vi "analysis_01(SubVI).vi"(8 "에러 입력(에러 없음)":errorcluster, 10 "품   번":string="034220", 11 "참조 번호 입력":T1 caption="client handle out") -> (0 "에러 출력":errorcluster, 1 "거래량":waveform(dbl)(graph), 2 "가격":waveform(i32)(graph), 3 "참조 번호 출력":T1 caption="client handle out", 5 "출력":T2)   [LabVIEW 2018]
uses:
  <vilib>/httpClient/ClientHandle.ctl
  <vilib>/httpClient/LabVIEWHTTPClient.lvlib
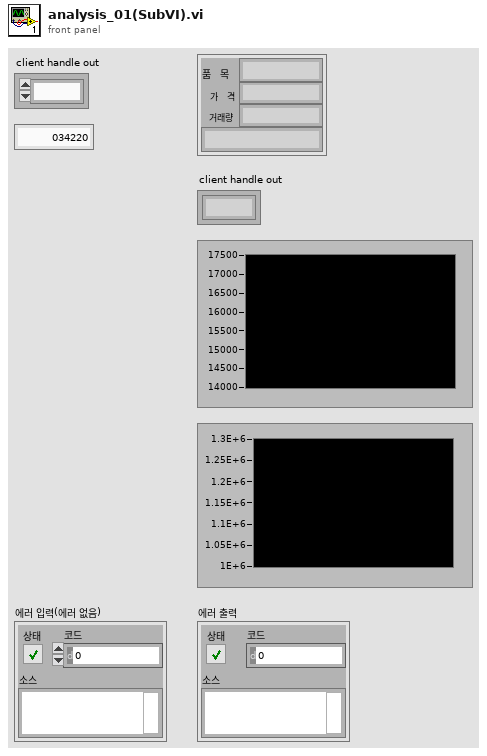
[diagram p1: front panel]
types:
  T1 = typedef "LabVIEWHTTPClient.lvlib/ClientHandle.ctl" = refnum<k1>
  T2 = cluster{"품   목":string, "가   격":i32, "거래량":dbl, "일시":string}
  T3 = cluster{"품목":string, "가격":i32, "거래량":dbl, "일시":string}
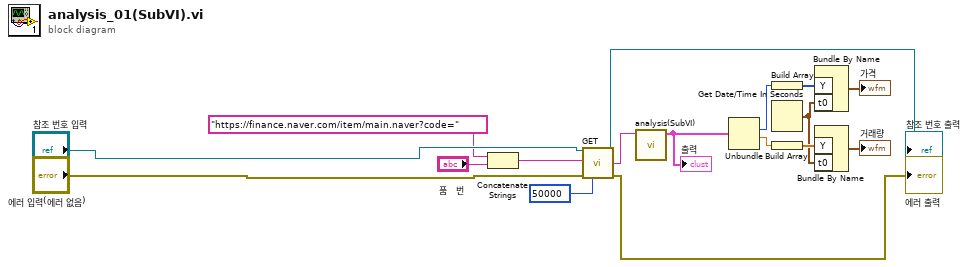
[diagram p0: block diagram]
diagram:
  n1 = Concatenate Strings("https://finance.naver.com/item/main.naver?code=" ("url"), "품   번") -> (w1:string)
  n2 = call <vilib>:"GET.vi"("client handle"="참조 번호 입력", "url"=w1, "error in (no error)"="에러 입력(에러 없음)", "timeout (10000)"=50000) -> ("client handle out"=→"참조 번호 출력":T1, "body"=w8:string, "error out"=→"에러 출력":errorcluster)  [unwired: 8 in, 1 out]
  n3 = call "analysis(SubVI).vi"("본문"=w8) -> ("출력"=w9:T3)  [unwired: 10 in]
  "출력" <- w9
  n4 = Unbundle(w9) -> ("가격"=w12:i32, "거래량"=w16:dbl)  [unwired: 2 out]
  n5 = Build Array(w12) -> (w10:i32[])
  n6 = Get Date/Time In Seconds() -> (seconds since 1Jan1904=w14:timestamp)
  n7 = Build Array(w16) -> (w15:dbl[])
  n8 = Bundle By Name("Y"=w10, "t0"=w14) -> (→"가격":waveform(i32))  [unwired: 1 in]
  n9 = Bundle By Name("Y"=w15, "t0"=w14) -> (→"거래량":waveform(dbl))  [unwired: 1 in]
